vi "UHR-Fleezers Control (host) -Leonardo 04-2018 V2.vi"(0 "Tab Control":T5(tab)=enum."Trap Control (RF)") -> ()   [LabVIEW 2013] (continued)
        n1860 = call-poly <vilib>:"Mean.vi"("X"=w2816) -> ("mean"=w2803:dbl)  [unwired: 1 out]
        n1861 = call-poly <vilib>:"Mean.vi"("X"=w2815) -> ("mean"=w2801:dbl)  [unwired: 1 out]
        n1862 = call-poly <vilib>:"Mean.vi"("X"=w2779) -> ("mean"=w2770:dbl)  [unwired: 1 out]
        n1863 = Subtract(x=w2874, y=w2866) -> (x-y=w2808:u64)
        n1864 = call-poly <vilib>:"Mean.vi"("X"=w2864) -> ("mean"=w2805:dbl)  [unwired: 1 out]
        n1865 = Initialize Array(1.0 ("element"), w2773) -> (w2769:dbl[])
        n1866 = Initialize Array(1.0 ("element"), w2808) -> (w2799:dbl[])
        n1867 = Multiply(x=w2769, y=w2770) -> (x*y=w2771:dbl[])
        n1868 = Multiply(x=w2799, y=w2801) -> (x*y=w2802:dbl[])
        n1869 = Multiply(x=w2799, y=w2803) -> (x*y=w2804:dbl[])
        n1870 = Multiply(x=w2799, y=w2798) -> (x*y=w2800:dbl[])
        n1871 = Multiply(x=w2799, y=w2805) -> (x*y=w2806:dbl[])
        n1872 = Build Array (concatenate)(w2814, w2800) -> (w2868:dbl[])
        n1873 = Build Array (concatenate)(w2816, w2804) -> (w2872:dbl[])
        n1874 = Build Array (concatenate)(w2815, w2802) -> (w2871:dbl[])
        n1875 = Build Array (concatenate)(w2779, w2771) -> (w2781:dbl[])
        n1876 = Build Array (concatenate)(w2864, w2806) -> (w2873:dbl[])
        n1877 = Reshape Array(w2868, w2752, w2751) -> (w2834:dbl[][])
        n1878 = Reshape Array(w2781, w2752, w2751) -> (w2777:dbl[][])
        n1879 = Reshape Array(w2872, w2752, w2751) -> (w2826:dbl[][])
        n1880 = Reshape Array(w2871, w2752, w2751) -> (w2841:dbl[][])
        n1881 = Reshape Array(w2873, w2752, w2751) -> (w2851:dbl[][])
        n1882 = Array Subset(array=w2841, index (col)=0 ("index"), length (col)=w2766) -> (w2846:dbl[][])  [unwired: 2 in]
        n1883 = Array Subset(array=w2841, index (col)=w2766) -> (w2844:dbl[][])  [unwired: 3 in]
        n1884 = Array Subset(array=w2826, index (col)=0 ("index"), length (col)=w2766) -> (w2832:dbl[][])  [unwired: 2 in]
        n1885 = Array Subset(array=w2826, index (col)=w2766) -> (w2830:dbl[][])  [unwired: 3 in]
        n1886 = Array Subset(array=w2777, index (col)=0 ("index"), length (col)=w2766) -> (w2776:dbl[][])  [unwired: 2 in]
        n1887 = Array Subset(array=w2777, index (col)=w2766) -> (w2774:dbl[][])  [unwired: 3 in]
        n1888 = Array Subset(array=w2851, index (col)=0 ("index"), length (col)=w2766) -> (w2850:dbl[][])  [unwired: 2 in]
        n1889 = Array Subset(array=w2851, index (col)=w2766) -> (w2848:dbl[][])  [unwired: 3 in]
        n1890 = Array Subset(array=w2834, index (col)=0 ("index"), length (col)=w2766) -> (w2839:dbl[][])  [unwired: 2 in]
        n1891 = Array Subset(array=w2834, index (col)=w2766) -> (w2837:dbl[][])  [unwired: 3 in]
        n1892 = for {
          tunnel: w2846 -> [w2888] mode=indexing
          tunnel: [w2887] -> w2845 mode=indexing
          workers-P: _ -> [_]
          n1893 = Reverse 1D Array(array=w2888) -> (reversed array=w2887:dbl[])
        }
        n1894 = for {
          tunnel: w2832 -> [w2884] mode=indexing
          tunnel: [w2883] -> w2831 mode=indexing
          workers-P: _ -> [_]
          n1895 = Reverse 1D Array(array=w2884) -> (reversed array=w2883:dbl[])
        }
        n1896 = for {
          tunnel: w2776 -> [w2882] mode=indexing
          tunnel: [w2881] -> w2775 mode=indexing
          workers-P: _ -> [_]
          n1897 = Reverse 1D Array(array=w2882) -> (reversed array=w2881:dbl[])
        }
        n1898 = for {
          tunnel: w2850 -> [w2890] mode=indexing
          tunnel: [w2889] -> w2849 mode=indexing
          workers-P: _ -> [_]
          n1899 = Reverse 1D Array(array=w2890) -> (reversed array=w2889:dbl[])
        }
        n1900 = for {
          tunnel: w2839 -> [w2886] mode=indexing
          tunnel: [w2885] -> w2838 mode=indexing
          workers-P: _ -> [_]
          n1901 = Reverse 1D Array(array=w2886) -> (reversed array=w2885:dbl[])
        }
        n1902 = Index Array(array=w2851, index (row)=0) -> (element=→"Waveform Graph":dbl[])  [unwired: 1 in]
        n1903 = Add(x=w2845, y=w2844) -> (x+y=w2843:dbl[][])
        n1904 = Add(x=w2831, y=w2830) -> (x+y=w2829:dbl[][])
        n1905 = Add(x=w2775, y=w2774) -> (x+y=w2759:dbl[][])
        n1906 = Add(x=w2849, y=w2848) -> (x+y=w2823:dbl[][])
        n1907 = Add(x=w2838, y=w2837) -> (x+y=w2836:dbl[][])
        n1908 = Divide(x=w2829, y=2) -> (x/y=w2827:dbl[][])
        n1909 = Divide(x=w2843, y=2) -> (x/y=w2788:dbl[][])
        n1910 = Divide(x=w2836, y=2) -> (x/y=w2790:dbl[][])
        n1911 = To Single Precision Float(number=w2823) -> (single precision float=w2822:sgl[][])
        n1912 = Transpose 2D Array(2D array=w2827) -> (transposed array=→"Data map":dbl[][])
        n1913 = To Single Precision Float(number=w2759) -> (single precision float=w2763:sgl[][])
        n1914 = To Single Precision Float(number=w2788) -> (single precision float=w2794:sgl[][])
        n1915 = To Single Precision Float(number=w2790) -> (single precision float=w2791:sgl[][])
        n1916 = call "IMAQ ArrayToImage"("Image Pixels (Float)"=w2822, "Image"=w2756) -> ("Image Out"=w2825:T3)  [unwired: 8 in, 1 out]
        n1917 = call "IMAQ ArrayToImage"("Image Pixels (Float)"=w2763, "Image"=w2755) -> ("Image Out"=w2765:T3)  [unwired: 8 in, 1 out]
        n1918 = call "IMAQ ArrayToImage"("Image Pixels (Float)"=w2794, "Image"=w2754) -> ("Image Out"=w2796:T3)  [unwired: 8 in, 1 out]
        n1919 = call "IMAQ ArrayToImage"("Image Pixels (Float)"=w2791, "Image"=w2753) -> ("Image Out"=w2793:T3)  [unwired: 8 in, 1 out]
        n1920 = call "IMAQ Symmetry"("Type of Symmetry"=w2824, "Image Src"=w2825) -> ("Image Dst Out"=w2820:T3)  [unwired: 3 in, 1 out]
        n1921 = call "IMAQ Symmetry"("Type of Symmetry"=w2764, "Image Src"=w2765) -> ("Image Dst Out"=w2761:T3)  [unwired: 3 in, 1 out]
        n1922 = call "IMAQ Symmetry"("Type of Symmetry"=w2795, "Image Src"=w2796) -> ("Image Dst Out"=→"Detection Laser X":T3)  [unwired: 3 in, 1 out]
        n1923 = call "IMAQ Symmetry"("Type of Symmetry"=w2792, "Image Src"=w2793) -> ("Image Dst Out"=→"Detection Laser Y":T3)  [unwired: 3 in, 1 out]
        n1924 = call "IMAQ Set Simple Calibration"("Calibration Axis Info"=T37 {"Origin Pixel"={"X"=0.0, "Y"=0.0}, "Angle Relative to Horizontal (deg)"=0.0, "Axis Reference"=0}, "Grid Descriptor"=T38 {"X Step"=0.3, "Y Step"=0.3, "Unit"=enum."Undefined"}, "Image"=w2820) -> ("Calibrated Image"=→"APD 1":T3)  [unwired: 7 in, 1 out]
        n1925 = call "IMAQ Set Simple Calibration"("Calibration Axis Info"=T37 {"Origin Pixel"={"X"=0.0, "Y"=0.0}, "Angle Relative to Horizontal (deg)"=0.0, "Axis Reference"=0}, "Grid Descriptor"=T38 {"X Step"=0.3, "Y Step"=0.3, "Unit"=enum."Undefined"}, "Image"=w2761) -> ("Calibrated Image"=→"APD 2":T3)  [unwired: 7 in, 1 out]
      }
    }
    n1926 = Subtract(x=w2303, y="APD 2 Offset") -> (x-y=w2300:waveform(dbl))
    n1927 = Subtract(x=w2305, y="APD 1 Offset") -> (x-y=w2301:waveform(dbl))
    n1928 = Index Array(array=w2320, index=3) -> (element=w2379:waveform(dbl))
    n1929 = Index Array(array=w2320, index=6) -> (element=w2376:waveform(dbl))
    n1930 = Build Array(w2301, w2300) -> (→"APD Chart":waveform(dbl)[])
    n1931 = Array Size(array=w2369) -> (size(s)=w2417:i32)
    n1932 = call <vilib>:"Std Deviation and Variance.vi"("X"=w2313) -> ("standard deviation"=w2312:dbl)  [unwired: 1 in, 2 out]
    n1933 = Add Array Elements(numeric array=w2313) -> (sum=w2315:u32)
    n1934 = Add Array Elements(numeric array=w2369) -> (sum=w2427:u32)
    n1935 = call <vilib>:"Std Deviation and Variance.vi"("X"=w2369) -> ("standard deviation"=w2368:dbl)  [unwired: 1 in, 2 out]
    n1936 = Divide(x=w2312, y=w2311) -> (x/y=w2308:dbl)
    "Rate sigma (Hz) 2" <- w2308
    n1937 = Multiply(x=w2311, y=w2417) -> (x*y=w2314:dbl)
    "Int. Time (s)" <- w2314
    n1938 = Divide(x=w2315, y=w2314) -> (x/y=w2309:dbl)
    "APD 2 Rate (Hz)" <- w2309
    n1939 = Divide(x=w2427, y=w2314) -> (x/y=w2366:dbl)
    "APD 1 Rate (Hz)" <- w2366
    n1940 = Divide(x=w2368, y=w2311) -> (x/y=w2367:dbl)
    "Rate sigma (Hz)" <- w2367
    n1941 = Divide(x=w2308, y=w2309) -> (x/y=→"Sigma/Mean 2":dbl)
    n1942 = Divide(x=w2367, y=w2366) -> (x/y=→"Sigma/Mean":dbl)
    n1943 = case shown="2" "Calibration" {
      tunnel: "T1 alpha_x (nm/V)" -> [_ w2719 w2740]
      tunnel: "T1 kappa_x (pN/nm)" -> [_ _ w2730]
      tunnel: "T2 alpha_x (nm/V)" -> [_ w2718 w2738]
      tunnel: "T2 kappa_x (pN/nm)" -> [_ _ w2731]
      tunnel: w2379 -> [w2701 w2716 w2736]
      tunnel: w2376 -> [w2700 w2714 w2734]
      tunnel: [w2701 w2713 w2733] -> w2169
      tunnel: [w2700 w2712 w2732] -> w2175
      tunnel: ["T1 X (V)" ("Label.Text") "T1 X (nm)" ("Label.Text") "T1 X (pN)" ("Label.Text")] -> w2397
      tunnel: ["T2 X (V)" ("Label.Text") "T2 X (nm)" ("Label.Text") "T2 X (pN)" ("Label.Text")] -> w2396
      tunnel: ["Position (V)" ("Label.Text") "Position (nm)" ("Label.Text") "Force (pN)" ("Label.Text")] -> w2398
      tunnel: w2378 -> [_ w2704 w2723]
      tunnel: w2380 -> [_ w2707 w2725]
      tunnel: ["Mean (V)" ("Label.Text") "Mean (nm)" ("Label.Text") "Mean (pN)" ("Label.Text")] -> w2393
      tunnel: ["Difference (V)" ("Label.Text") "Difference (nm)" ("Label.Text") "Difference (pN)" ("Label.Text")] -> w2328
      frame 0, Default {
      }
      frame 1 {
        # "position"
        n1944 = Unbundle By Name(w2716) -> ("Y"=w2720:dbl[])
        n1945 = Unbundle By Name(w2714) -> ("Y"=w2705:dbl[])
        n1946 = Subtract(x=w2720, y=w2707) -> (x-y=w2708:dbl[])
        n1947 = Subtract(x=w2705, y=w2704) -> (x-y=w2706:dbl[])
        n1948 = Multiply(x=w2706, y=w2718) -> (x*y=w2715:dbl[])
        n1949 = Multiply(x=w2719, y=w2708) -> (x*y=w2717:dbl[])
        n1950 = Bundle By Name(cluster=w2714, "Y"=w2715) -> (w2712:waveform(dbl))
        n1951 = Bundle By Name(cluster=w2716, "Y"=w2717) -> (w2713:waveform(dbl))
      }
      frame 2 {
        # "force"
        n1952 = Unbundle By Name(w2736) -> ("Y"=w2741:dbl[])
        n1953 = Unbundle By Name(w2734) -> ("Y"=w2739:dbl[])
        n1954 = Subtract(x=w2739, y=w2723) -> (x-y=w2724:dbl[])
        n1955 = Subtract(x=w2741, y=w2725) -> (x-y=w2726:dbl[])
        n1956 = Compound Arithmetic op=MULTIPLY(w2724, w2738, w2731) -> (w2735:dbl[])
        n1957 = Compound Arithmetic op=MULTIPLY(w2730, w2740, w2726) -> (w2737:dbl[])
        n1958 = Bundle By Name(cluster=w2734, "Y"=w2735) -> (w2732:waveform(dbl))
        n1959 = Bundle By Name(cluster=w2736, "Y"=w2737) -> (w2733:waveform(dbl))
      }
    }
    n1960 = feedback-in #17("Calibration") -> ()
    n1961 = feedback #17(u16 1 ("Calibration")) -> (w2400:u16)
    n1962 = local read "Trap 2 Bead Size (nm)"() -> (w2208:dbl)
    n1963 = local read "Trap 1 Bead Size (nm)"() -> (w2207:dbl)
    n1964 = local read "AOM X Cal (nm/MHz)"() -> (w2205:dbl)
    n1965 = local read "Trap Delta (MHz)"() -> (w2204:dbl)
    n1966 = Not Equal?(x=w2400, y="Calibration") -> (x != y?=w2357:bool)
    n1967 = Multiply(x=w2205, y=w2204) -> (x*y=w2209:dbl)
    n1968 = Unbundle By Name(w2169) -> ("Y"=w2174:dbl[])
    n1969 = Unbundle By Name(w2175) -> ("Y"=w2173:dbl[])
    n1970 = Add(x=w2208, y=w2207) -> (x+y=w2211:dbl)
    n1971 = case shown="False" "Negate trap 2 force" {
      tunnel: [-1.0 1.0] -> w2386
      frame False {
      }
      frame True {
      }
    }
    n1972 = Unbundle By Name(w2379) -> ("Y"=w2382:dbl[])
    n1973 = Unbundle By Name(w2376) -> ("Y"=w2385:dbl[])
    n1974 = Divide(x=w2211, y=2.0) -> (x/y=w2206:dbl)
    n1975 = Subtract(x=w2174, y=w2173) -> (x-y=w2171:dbl[])
    n1976 = Subtract(x=w2382, y=w2380) -> (x-y=w2383:dbl[])
    n1977 = Subtract(x=w2385, y=w2378) -> (x-y=w2384:dbl[])
    n1978 = Divide(x=w2171, y=2.0) -> (x/y=w2170:dbl[])
    n1979 = Multiply(x=w2384, y="T2 alpha_x (nm/V)") -> (x*y=w2375:dbl[])
    n1980 = Multiply(x="T1 alpha_x (nm/V)", y=w2383) -> (x*y=w2374:dbl[])
    n1981 = Multiply(x=w2175, y=w2386) -> (x*y=w2387:waveform(dbl))
    n1982 = Bundle By Name(cluster=w2169, "Y"=w2170) -> (w2168:waveform(dbl))
    n1983 = case shown="True" "Read Lateness and Rel Phase" {
      tunnel: w2181 -> [w2665 w2689]
      tunnel: w2220 -> [w2666 w2688]
      tunnel: [w2665 w2687] -> w2372
      tunnel: [w2666 w2686] -> w2371
      frame False {
      }
      frame True {
        n1984 = xnode "Read/Write Control"("FPGA VI Reference In"=w2689, "error in"=w2688) -> ("FPGA VI Reference Out"=w2687:T20, "error out"=w2686:errorcluster, "GI Relative phase"=→"GI relative phase":i16, "Relative phase"=→"Relative phase (AI1)":i16, "AI Late Counter"=→"Late Counter (AI1)":u8, "GI Late Counter"=→"GI Late Counter":u8, "MCL Late Counter"=→"MCL Late Counter":u8, "MCL Relative Phase"=→"Relative Phase (MCL)":i16, "APD Acq Relative Phase"=→"APD Acq Relative Phase":i16, "APD 1 Gate Relative Phase"=→"APD 1 Gate Relative Phase":i16, "APD Acq Late Counter"=→"APD Acq Late Counter":u16, "APD 1 Gate Late Counter"=→"APD 1 Gate Late Counter":u8, "Green FB Relative Phase"=→"Relative phase (Green FB)":i16, "GI Relative phase"=→"GI relative phase 2":i16, "GI Late Counter 2"=→"GI Late Counter 2":u16, "Trap Pos FIFO Timeout"=→"Trap Pos FIFO Timeout":u16, "Trap AI FIFO Timeout"=→"Trap AI FIFO Timeout":u16, "APD 1 Counts 0"=→"APD1 counts 1":u32, "APD 1 Counts 1"=→"APD1 counts 2":u32, "APD 2 Counts 0"=→"APD2 counts 1":u32, "APD 2 Counts 1"=→"APD2 counts 2":u32)
      }
    }
    n1985 = Subtract(x=w2375, y=w2374) -> (x-y=w2203:dbl[])
    n1986 = call-poly <vilib>:"Mean.vi"("X"=w2203) -> ("mean"=w2210:dbl)  [unwired: 1 out]
    n1987 = Add(x=w2209, y=w2210) -> (x+y=w2213:dbl)
    n1988 = Subtract(x=w2213, y=w2206) -> (x-y=→"Tether Extension (nm, calculated)":dbl)
    n1989 = Unbundle By Name(w2175) -> ("Y"=w2166:dbl[])
    n1990 = Unbundle By Name(w2169) -> ("Y"=w2167:dbl[])
    n1991 = Build Array(w2169, w2387, w2168) -> (→"Force":waveform(dbl)[])
    n1992 = Subtract(x=w2203, y="Offset (nm)") -> (x-y=w2347:dbl[])
    n1993 = call-poly <vilib>:"Mean.vi"("X"=w2166) -> ("mean"=w2164:dbl)  [unwired: 1 out]
    "T2 X" <- w2164
    n1994 = call-poly <vilib>:"Mean.vi"("X"=w2167) -> ("mean"=w2165:dbl)  [unwired: 1 out]
    "T1 X" <- w2165
    n1995 = Subtract(x=w2167, y=w2166) -> (x-y=w2349:dbl[])
    n1996 = Bundle By Name(cluster=w2379, "Y"=w2347) -> (w2319:waveform(dbl))
    "Bead Separation" <- w2319
    n1997 = Divide(x=w2349, y=2.0) -> (x/y=→"Vec Mean of T1 T2":dbl[])
    n1998 = case shown="True" w2357 {
      tunnel: w2398 -> [_ w2694]
      tunnel: w2397 -> [_ w2693]
      tunnel: w2396 -> [_ w2692]
      tunnel: w2393 -> [_ w2691]
      tunnel: w2328 -> [_ w2690]
      frame False {
      }
      frame True {
        n1999 = property on="Force" class="WFChart (strict)"("YScale.NameLbl.Text"=w2694) -> ()  [unwired: 2 in, 2 out]
        n2000 = property on="T2 X" class="DigNum (strict)"("Caption.Text"=w2692) -> ()  [unwired: 2 in, 2 out]
        n2001 = property on="T1 X" class="DigNum (strict)"("Caption.Text"=w2693) -> ()  [unwired: 2 in, 2 out]
        n2002 = property on="Mean" class="DigNum (strict)"("Caption.Text"=w2691) -> ()  [unwired: 2 in, 2 out]
        n2003 = property on="Difference" class="DigNum (strict)"("Caption.Text"=w2690) -> ()  [unwired: 2 in, 2 out]
      }
    }
    n2004 = local read "Tether"() -> (w2351:bool)
    n2005 = Subtract(x=w2165, y=w2164) -> (x-y=w2395:dbl)
    n2006 = Add(x=w2165, y=w2164) -> (x+y=→"Difference":dbl)
    n2007 = feedback #18(w2347) -> (w2346:dbl[])
    n2008 = Divide(x=w2395, y=2.0) -> (x/y=w2178:dbl)
    "Mean" <- w2178
    n2009 = case shown="True" w2351 {
      tunnel: w2178 -> [_ w2624]
      frame False {
      }
      frame True {
        n2010 = Greater?(x="Lost Tether Alarm Threshold (pN)", y=w2624) -> (0:w2622:bool)
        n2011 = case shown="True" w2622 {
          frame False {
          }
          frame True {
            n2012 = flat-sequence {
              frame #0 {
                # "stop only if saving"
                n2013 = local read "Saving..."() -> (w2637:bool)
                n2014 = And(x=w2637, y="TA Cancel Save?") -> (x .and. y?=w2636:bool)
                n2015 = local write "Stop Saving"(w2636) -> ()
              }
              frame #1 {
                n2016 = case shown="True" "TA Green Off?" {
                  frame False {
                  }
                  frame True {
                    w2640 = FALSE ("Fl. Triggered...")
                    n2017 = local write "Fl. Triggered..."(w2640) -> ()
                    n2018 = property on="Green Laser ON/Interlacing" class="Bool (strict)"("Val(Sgnl)"=w2640) -> ()  [unwired: 2 in, 2 out]
                  }
                }
              }
            }
            n2019 = local read "Time tether formed"() -> (w2631:timestamp)
            n2020 = Get Date/Time In Seconds() -> (seconds since 1Jan1904=w2632:timestamp)
            n2021 = Subtract(x=w2632, y=w2631) -> (x-y=w2630:dbl)
            n2022 = Number To Decimal String(number=w2630) -> (decimal integer string=w2627:string)  [unwired: 1 out]
            n2023 = local read "Messages"() -> (w2634:string)
            n2024 = call <vilib>:"Beep.vi"() -> ()  [unwired: 3 in, 9 out]
            n2025 = Concatenate Strings("Lost tether (" ("Message to add"), w2627, " s)." ("string")) -> (w2629:string)
            n2026 = local write "Tether"(FALSE ("Tether")) -> ()
            n2027 = call "Update messages.vi"("Message to add"=w2629, "Old message string"=w2634) -> ("New message string"=w2633:string)
            n2028 = local write "Messages"(w2633) -> ()
            n2029 = property on="Trap Pos. FB ON" class="Bool (strict)"("Val(Sgnl)"=FALSE ("Value (Signaling)")) -> ()  [unwired: 2 in, 2 out]
          }
        }
      }
    }
    n2030 = Build Array (concatenate)(w2347, w2346) -> (w2345:dbl[])
    n2031 = Split 1D Array(array=w2345, index=w2231) -> (first subarray=w2341:dbl[])  [unwired: 1 out]
    n2032 = feedback-in #18(w2341) -> ()
    n2033 = call-poly <vilib>:"Mean.vi"("X"=w2341) -> ("mean"=w2340:dbl)  [unwired: 1 out]
    "Bead Mean (nm)" <- w2340
    n2034 = Subtract(x=w2341, y=w2340) -> (x-y=w2339:dbl[])
    n2035 = Square(x=w2339) -> (x^2=w2338:dbl[])
    n2036 = call-poly <vilib>:"Mean.vi"("X"=w2338) -> ("mean"=w2337:dbl)  [unwired: 1 out]
    n2037 = case shown="True" "Semi Passive ON" {
      tunnel: "Semi Passive mode" -> [_ w2505]
      tunnel: "Jump Force (pN)" -> [_ w2504]
      tunnel: w2178 -> [_ w2503]
      frame False {
      }
      frame True {
        n2038 = case shown="\"Use Feedback\"" w2505 {
          tunnel: w2504 -> [_ w2508 w2524]
          tunnel: w2503 -> [_ w2507 w2523]
          frame "None" {
          }
          frame "Use Feedback" {
            n2039 = local read "Target Force (pN)"() -> (w2510:dbl)
            n2040 = Less?(x=w2508, y=w2510) -> (x < y?=w2509:bool)
            n2041 = case shown="True" w2509 {
              tunnel: w2508 -> [w2517 w2520]
              tunnel: w2507 -> [w2516 w2519]
              tunnel: [w2515 w2518] -> w2506
              frame False {
                n2042 = Less?(x=w2517, y=w2516) -> (x < y?=w2515:bool)
              }
              frame True {
                n2043 = Greater?(x=w2520, y=w2519) -> (0:w2518:bool)
              }
            }
            n2044 = case shown="True" w2506 {
              frame False {
                n2045 = local read "Trap Pos. FB ON"() -> (w2511:bool)
                n2046 = case shown="True" w2511 {
                  frame False {
                  }
                  frame True {
                    n2047 = property on="Trap Pos. FB ON" class="Bool (strict)"("Val(Sgnl)"=FALSE) -> ()  [unwired: 2 in, 2 out]
                  }
                }
              }
              frame True {
                n2048 = local read "Trap Pos. FB ON"() -> (w2513:bool)
                n2049 = case shown="False" w2513 {
                  frame False {
                    n2050 = property on="Trap Pos. FB ON" class="Bool (strict)"("Val(Sgnl)"=TRUE) -> ()  [unwired: 2 in, 2 out]
                  }
                  frame True {
                  }
                }
              }
            }
          }
          frame "Sharp Jump" {
            n2051 = local read "Target Force (pN)"() -> (w2526:dbl)
            n2052 = Greater?(x=w2524, y=w2526) -> (0:w2525:bool)
            n2053 = case shown="True" w2525 {
              tunnel: w2524 -> [w2541 w2545]
              tunnel: w2523 -> [w2542 w2544]
              tunnel: [w2540 w2543] -> w2522
              frame False {
                n2054 = Greater?(x=w2542, y=w2541) -> (0:w2540:bool)
              }
              frame True {
                n2055 = Less?(x=w2545, y=w2544) -> (x < y?=w2543:bool)
              }
            }
            n2056 = Subtract(x=w2524, y=w2526) -> (x-y=w2521:dbl)
            n2057 = case shown="True" w2522 {
              tunnel: w2521 -> [_ w2532]
              frame False {
              }
              frame True {
                n2058 = local read "T1 kappa_x (pN/nm)"() -> (w2537:dbl)
                n2059 = local read "T2 kappa_x (pN/nm)"() -> (w2538:dbl)
                n2060 = Reciprocal(x="DNA stiffness (pN / nm)") -> (1/x=w2534:dbl)
                n2061 = Reciprocal(x=w2537) -> (1/x=w2536:dbl)
                n2062 = Reciprocal(x=w2538) -> (1/x=w2535:dbl)
                n2063 = Compound Arithmetic op=ADD(w2536, w2535, w2534) -> (w2533:dbl)
                n2064 = local read "AOM X Cal (nm/MHz)"() -> (w2531:dbl)
                n2065 = Multiply(x=w2533, y=w2532) -> (x*y=w2530:dbl)
                n2066 = local read "Trap Delta (MHz)"() -> (w2528:dbl)
                n2067 = Divide(x=w2530, y=w2531) -> (x/y=w2529:dbl)
                n2068 = Subtract(x=w2528, y=w2529) -> (x-y=w2527:dbl)
                n2069 = property on="Trap Delta (MHz)" class="DigNum (strict)"("Val(Sgnl)"=w2527) -> ()  [unwired: 2 in, 2 out]
              }
            }
          }
        }
      }
    }
    n2070 = Square Root(x=w2337) -> (sqrt(x)=w2336:dbl)
    n2071 = Multiply(x=10.0, y=w2336) -> (x*y=→"RMS (Ang)":dbl)
    n2072 = xnode "Read/Write Control"("FPGA VI Reference In"=w2372, "error in"=w2371) -> ("FPGA VI Reference Out"=w2481:T20, "error out"=w2475:errorcluster, "AI2 Y Sum Set 1"=w2471:i16, "AI2 Y Sum Set 2"=w2470:i16, "AI1 X Set 1"=w2265:fxp<+/-,16,1>, "AI1 X Set 2"=w2264:fxp<+/-,16,1>, "Trap Pos FB Int Signal"=→"Trap Pos FB Int Signal":fxp<+/-,24,9>, "Trap Pos FB Int-Norm Signal"=→"Trap Pos FB Int-Norm Signal":fxp<+/-,16,1>, "Trap Pos FB Action"=w2258:i64, "Scanning"=→"AOD Scanning":bool, "Scan I"=→"AOD Scan I":u64, "Scanning MCL"=w2473:bool, "Scan I (MCL)"=→"MCL Scan I":u64, "Green FB Signals"=w2412:T48, "BD1 amplitude 1 out"=w2163:u16, "BD1 amplitude 2 out"=w2148:u16)  [unwired: 1 out]
    "MCL Scanning" <- w2473
    "Trap Pos FB Action" <- w2258
    n2073 = local read "AI2 (V)"() -> (w2472:cluster{"Set 1":dbl, "Set 2":dbl})
    n2074 = Bundle By Name(cluster=w2472, "Set 1"=w2471, "Set 2"=w2470) -> (w2468:cluster{"Set 1":dbl, "Set 2":dbl})
    n2075 = Divide(x=w2258, y=327.67) -> (x/y=→"Action (%)":dbl)
    n2076 = local read "Trap X (AI1)"() -> (w2278:T1)
    n2077 = Divide(x=w2468, y=3276.7) -> (x/y=w2467:cluster{"Set 1":dbl, "Set 2":dbl})
    n2078 = local write "AI2 (V)"(w2467) -> ()
    n2079 = Bundle(cluster=w2278, "Trap 1"=w2265, "Trap 2"=w2264) -> (→"Trap X (AI1)":T1)
    n2080 = Scale By Power Of 2(n=i16 12, x=ext 1.0) -> (x*2^n=w2159:ext)
    n2081 = Subtract(x=w2159, y=ext 1.0) -> (x-y=w2156:ext)
    n2082 = Divide(x=w2412, y=3276.7) -> (x/y=w2408:T49)
    n2083 = Multiply(x=w2163, y=ext 100.0) -> (x*y=w2157:ext)
    n2084 = Unbundle By Name(w2408) -> ("Green FB Ch 0"=w2411:dbl, "Green FB Ch 1"=w2410:dbl, "Green FB Ch 2"=w2409:dbl)
    n2085 = local read "All FB On/Off"() -> (w2147:bool)
    n2086 = Divide(x=w2157, y=w2156) -> (x/y=w2146:ext)
    "Trap 1 amplitude" <- w2146
    n2087 = Scale By Power Of 2(n=i16 12, x=ext 1.0) -> (x*2^n=w2152:ext)
    n2088 = Subtract(x=w2152, y=ext 1.0) -> (x-y=w2155:ext)
    n2089 = Multiply(x=w2148, y=ext 100.0) -> (x*y=w2154:ext)
    n2090 = Divide(x=w2411, y=w2409) -> (x/y=w2407:dbl)
    n2091 = Divide(x=w2410, y=w2409) -> (x/y=w2406:dbl)
    n2092 = flat-sequence "To save data" {
      tunnel: [w3521] -> w2492
      tunnel: [w3522] -> w2491
      tunnel: w2443 -> [w3515]
      tunnel: w2343 -> [w3519]
      tunnel: ["Save Calibration"] -> w2464
      tunnel: w2461 -> [w3518]
      tunnel: [w3511] -> w2460
      tunnel: [w3508] -> w2459
      tunnel: [w3505] -> w2458
      tunnel: w2442 -> [w3507]
      tunnel: w2355 -> [w3501]
      tunnel: [w3501] -> w2354
      tunnel: ["Start Saving"] -> w2321
      tunnel: [w3495] -> w2247
      tunnel: [w3494] -> w2246
      tunnel: w2492 -> [w3756]
      tunnel: w2491 -> [w3755]
      tunnel: w2248 -> [w3754]
      tunnel: w2464 -> [w3753]
      tunnel: w2460 -> [w3751]
      tunnel: w2459 -> [w3750]
      tunnel: w2458 -> [w3749]
      tunnel: w2330 -> [w3748]
      tunnel: w2364 -> [w3747]
      tunnel: w2354 -> [w3746]
      tunnel: w2321 -> [w3745]
      tunnel: w2319 -> [w3744]
      tunnel: w2295 -> [w3743]
      tunnel: w2247 -> [w3742]
      tunnel: w2246 -> [w3741]
      tunnel: w2245 -> [w3740]
      frame #0 {
        n2093 = Or(x="Save N Sets", y="Start Saving") -> (x .or. y?=w3502:bool)
        n2094 = To Double Precision Float(number=w3518) -> (double precision float=w3512:dbl)
        n2095 = Build Array(w3502, "Save Calibration", w3515, w3507) -> (w3517:bool[])
        n2096 = Compound Arithmetic op=OR("Save Calibration", w3515, w3502, w3507) -> (w3520:bool)
        n2097 = Boolean Array To Number(Boolean array=w3517) -> (number=w3514:u32)
        n2098 = feedback #19(FALSE ("Save APD Data\nwith Trap Data")) -> (w3496:bool)
        n2099 = feedback #20(refnum<k0> refnum) -> (w3523:refnum<file>)
        n2100 = feedback #21(refnum<k0> refnum) -> (w3498:refnum<file>)
        n2101 = feedback #22(FALSE ("Save APD Data\nwith Trap Data")) -> (w3506:bool)
        n2102 = feedback #23(refnum<k0> refnum) -> (w3509:refnum<file>)
        n2103 = feedback #24(0) -> (w3525:i32)
        n2104 = feedback #25() -> (w3513:u32)  [unwired: 1 out]
        n2105 = case shown="True" w3520 {
          tunnel: [w3532 1] -> w3521
          tunnel: w3525 -> [w3534 _]
          tunnel: [w3533 w3552] -> w3522
          tunnel: w3523 -> [w3533 _]
          tunnel: w3519 -> [_ w3572]
          tunnel: w3512 -> [_ w3570]
          tunnel: w3514 -> [_ w3573]
          tunnel: [w3531 w3551] -> w3511
          tunnel: w3513 -> [w3531 _]
          tunnel: [w3530 w3549] -> w3508
          tunnel: w3509 -> [w3530 _]
          tunnel: [w3529 w3548] -> w3505
          tunnel: w3506 -> [w3529 _]
          tunnel: "Start Saving" -> [_ w3546]
          tunnel: w3501 -> [_ w3545]
          tunnel: [w3528 w3536] -> w3494
          tunnel: w3498 -> [w3528 _]
          tunnel: [w3527 w3535] -> w3495
          tunnel: w3496 -> [w3527 _]
          frame False {
            n2106 = Increment(x=w3534) -> (x+1=w3532:i32)
          }
          frame True {
            w3542 = FALSE ("Start Saving")
            w3547 = 9.0  # File Version
            w3555 = FALSE ("prepend array or string size? (T)")
            w3553 = T30."big-endian, network order" ("byte order (0:big-endian, network order)")
            # "write file headers"
            n2107 = local read "BD 1 Frequency 1 (MHz)"() -> (w3569:dbl)
            n2108 = local read "BD 2 Frequency 1 (MHz)"() -> (w3568:dbl)
            n2109 = local read "BD 1 Frequency 2 (MHz)"() -> (w3567:dbl)
            n2110 = local read "BD 2 Frequency 2 (MHz)"() -> (w3566:dbl)
            n2111 = local read "BD 1 Frequency 3 (MHz)"() -> (w3565:dbl)
            n2112 = local read "BD 2 Frequency 3 (MHz)"() -> (w3564:dbl)
            n2113 = Array Size(array=w3545) -> (size(s)=w3544:i32)
            n2114 = To Double Precision Float(number=w3544) -> (double precision float=w3543:dbl)
            n2115 = local write "Save Calibration"(w3542) -> ()
            n2116 = local write "Start Saving"(w3542) -> ()
            n2117 = Build Array("Save APD Data\nwith Trap Data", "Save Trap Pos. Data") -> (w3539:bool[])
            n2118 = Boolean Array To Number(Boolean array=w3539) -> (number=w3538:u32)
            n2119 = Build Array(w3569, w3568, w3567, w3566, w3565, w3564) -> (w3563:dbl[])
            n2120 = case shown="4" w3573 {
              tunnel: w3572 -> [w3644 w3664 w3680 w3718]
              tunnel: w3543 -> [w3649 w3671 w3700 w3737]
              tunnel: w3570 -> [w3648 w3670 w3699 w3736]
              tunnel: [w3645 w3666 w3691 w3728] -> w3561
              tunnel: [w3636 "Cal sets to save" w3681 w3719] -> w3551
              tunnel: w3563 -> [w3646 w3667 w3693 w3730]
              tunnel: "Save APD Data\nwith Trap Data" -> [w3643 _ w3677 w3716]
              tunnel: [w3643 w3658 w3677 w3716] -> w3548
              tunnel: w3547 -> [w3639 w3659 w3675 w3714]
              tunnel: w3546 -> [w3638 _ _ _]
              tunnel: [w3629 w3658 w3674 w3704] -> w3535
              tunnel: "Save Trap Pos. Data" -> [w3629 _ w3674 w3704]
              tunnel: w3538 -> [w3628 _ w3673 w3703]
              frame 1, Default {
                # "timeseries"
                n2121 = case shown="True" "Profile" {
                  tunnel: [w3652 w3655] -> w3633
                  tunnel: [w3652 w3654] -> w3632
                  tunnel: [w3652 w3653] -> w3631
                  tunnel: [w3652 w3657] -> w3630
                  frame False {
                    w3652 = 0.0 ("f")
                  }
                  frame True {
                    n2122 = local read "Current Position"() -> (w3656:dbl[])
                    n2123 = local read "Y change (mm)"() -> (w3657:dbl)
                    n2124 = call "subVI_explode3array.vi"("Array"=w3656) -> ("x"=w3655:dbl, "y"=w3654:dbl, "z"=w3653:dbl)  [unwired: 12 in]
                  }
                }
                n2125 = local read "Save ave N"() -> (w3651:dbl)
                n2126 = Multiply(x=w3651, y=w3644) -> (x*y=w3650:dbl)
                n2127 = To Double Precision Float(number=w3628) -> (double precision float=w3642:dbl)
                n2128 = Build Array(w3639, w3644, w3650, w3649, w3648, 0.0 ("f")) -> (w3647:dbl[])
                n2129 = Build Array(w3642, w3633, w3632, w3631, w3630) -> (w3640:dbl[])
                n2130 = Select(t=u32 4000000000, s=w3638, f="N sets to save") -> (s? t:f=w3636:u32)
                n2131 = Build Array (concatenate)(w3647, w3646, w3640) -> (w3645:dbl[])
              }
              frame 2 {
                w3661 = 0.0 ("f")
                w3658 = FALSE ("Save APD Data\nwith Trap Data")
                # "calibration"
                n2132 = Boolean To (0,1)(Boolean=w3658) -> (0, 1=w3663:i16)
                n2133 = To Double Precision Float(number=w3663) -> (double precision float=w3662:dbl)
                n2134 = Build Array(w3662, w3661, w3661, w3661, w3661) -> (w3660:dbl[])
                n2135 = Build Array(w3659, w3664, w3664, w3671, w3670, 1.0 ("t")) -> (w3668:dbl[])
                n2136 = Build Array (concatenate)(w3668, w3667, w3660) -> (w3666:dbl[])
                "Calibrating Trap..." <- TRUE ("Calibrating...")
              }
              frame 4 {
                w3678 = 0.0 ("f")
                # "write file header for a trap \nraster scan"
                # "scan dir (x/y = 0/1)"
                # "cycles/step"
                # "n scans (f/b)"
                # "steps"
                # "freq. range"
                # "AOD raster scan"
                n2137 = local read "Number of F/B Scans (AOD)"() -> (w3685:u16)
                n2138 = local read "Cycles/step (AOD)"() -> (w3687:u64)
                n2139 = local read "Scan Range (MHz)"() -> (w3690:dbl)
                n2140 = local read "Scan steps (AOD)"() -> (w3689:u64)
                n2141 = local read "Scan BD"() -> (w3697:bool)
                n2142 = local read "Save ave N"() -> (w3702:dbl)
                n2143 = Boolean To (0,1)(Boolean=w3697) -> (0, 1=w3696:i16)
                n2144 = To Double Precision Float(number=w3685) -> (double precision float=w3684:dbl)
                n2145 = To Double Precision Float(number=w3689) -> (double precision float=w3688:dbl)
                n2146 = To Double Precision Float(number=w3687) -> (double precision float=w3686:dbl)
                n2147 = To Double Precision Float(number=w3696) -> (double precision float=w3695:dbl)
                n2148 = Multiply(x=w3702, y=w3680) -> (x*y=w3701:dbl)
                n2149 = To Double Precision Float(number=w3673) -> (double precision float=w3679:dbl)
                n2150 = Build Array(w3679, w3678, w3678, w3678, w3678) -> (w3676:dbl[])
                n2151 = local read "N sets should be saved"() -> (w3682:dbl)
                n2152 = Build Array(w3695, w3690, w3688, w3686, w3684) -> (w3692:dbl[])
                n2153 = Build Array(w3675, w3680, w3701, w3700, w3699, 2.0 ("t")) -> (w3694:dbl[])
                n2154 = Round Toward +Infinity(x=w3682) -> (ceil(x): smallest int >= x=w3683:dbl)
                n2155 = Build Array (concatenate)(w3694, w3693, w3676, w3692) -> (w3691:dbl[])
                n2156 = To Unsigned Long Integer(number=w3683) -> (unsigned 32bit integer=w3681:u32)
              }
              frame 8 {
                w3711 = 0.0 ("f")
                # "MCL raster scan"
                n2157 = local read "Number of scans (MCL)"() -> (w3706:u64)
                n2158 = local read "Scan lines (y)"() -> (w3705:u64)
                n2159 = local read "2D or 1D Scan"() -> (w3708:bool)
                n2160 = local read "Scan Range (V)\n(of steps)"() -> (w3727:dbl)
                n2161 = local read "Fast Scan Dir"() -> (w3734:bool)
                n2162 = local read "Cycles/step (MCL)"() -> (w3724:u64)
                n2163 = local read "Scan steps (MCL)"() -> (w3726:u64)
                n2164 = Select(t=w3705, s=w3708, f=w3706) -> (s? t:f=w3707:u64)
                n2165 = Boolean To (0,1)(Boolean=w3708) -> (0, 1=w3710:i16)
                n2166 = local read "Save ave N"() -> (w3739:dbl)
                n2167 = local read "Initial X"() -> (w3713:dbl)
                n2168 = local read "Initial Y"() -> (w3712:dbl)
                n2169 = To Double Precision Float(number=w3710) -> (double precision float=w3709:dbl)
                n2170 = Boolean To (0,1)(Boolean=w3734) -> (0, 1=w3733:i16)
                n2171 = To Double Precision Float(number=w3707) -> (double precision float=w3722:dbl)
                n2172 = To Double Precision Float(number=w3726) -> (double precision float=w3725:dbl)
                n2173 = To Double Precision Float(number=w3724) -> (double precision float=w3723:dbl)
                n2174 = To Double Precision Float(number=w3733) -> (double precision float=w3732:dbl)
                n2175 = Multiply(x=w3739, y=w3718) -> (x*y=w3738:dbl)
                n2176 = To Double Precision Float(number=w3703) -> (double precision float=w3717:dbl)
                n2177 = local read "N sets should be saved (MCL)"() -> (w3720:dbl)
                n2178 = Build Array(w3717, w3709, w3711, w3711, w3711) -> (w3715:dbl[])
                n2179 = Build Array(w3732, w3727, w3725, w3723, w3722, w3713, w3712) -> (w3729:dbl[])
                n2180 = Build Array(w3714, w3718, w3738, w3737, w3736, 3.0 ("t")) -> (w3731:dbl[])
                n2181 = Round Toward +Infinity(x=w3720) -> (ceil(x): smallest int >= x=w3721:dbl)
                n2182 = Build Array (concatenate)(w3731, w3730, w3715, w3729) -> (w3728:dbl[])
                n2183 = To Unsigned Long Integer(number=w3721) -> (unsigned 32bit integer=w3719:u32)
              }
            }
            n2184 = local read "Index"() -> (w3578:dbl)
            n2185 = call "Create new save file.vi"("Insert"="", "Ext"=".dat", "Index In"=w3578) -> ("Path Out"=w3537:path, "Index Out"=w3550:dbl)
            n2186 = local write "Save file name"(w3537) -> ()
            n2187 = local write "Index"(w3550) -> ()
            n2188 = local write "Save index"(w3550) -> ()
            n2189 = Array Size(array=w3561) -> (size(s)=w3562:i32)
            n2190 = Open/Create/Replace File(file path (use dialog)=w3537, operation (0:open)=T24."create", access (0:read/write)=enum16{"read/write", "read-only", "write-only"}."write-only") -> (refnum out=w3575:refnum<file>)  [unwired: 1 in, 4 out]
            n2191 = local write "Saving..."(TRUE ("Saving...")) -> ()
            n2192 = To Double Precision Float(number=w3562) -> (double precision float=w3560:dbl)
            n2193 = String Length(string="Comment (data description)") -> (length=w3558:i32)
            n2194 = To Double Precision Float(number=w3558) -> (double precision float=w3557:dbl)
            n2195 = Deny Access(7:w3575) -> (3:w3574:refnum<file>)  [unwired: 1 in, 2 out]
            n2196 = Build Array (concatenate)(w3560, w3561, w3557) -> (w3559:dbl[])
            n2197 = case "If fluorescence data to be saved" shown="True" w3548 {
              tunnel: w3537 -> [_ w3627]
              tunnel: [refnum<k0> refnum w3607] -> w3549
              frame False {
              }
              frame True {
                w3606 = 0.0
                n2198 = local read "APD Integration Time (s)"() -> (w3612:dbl)
                n2199 = local read "N APD Samp/step"() -> (w3605:dbl)
                n2200 = Path To String(path=w3627) -> (string=w3626:string)
                n2201 = String Length(string=w3626) -> (length=w3625:i32)
                n2202 = Subtract(x=w3625, y=4) -> (x-y=w3623:i32)
                n2203 = String Subset(string=w3626, length (rest)=w3623) -> (substring=w3622:string)  [unwired: 1 out]
                n2204 = Build Array(w3612, w3605, w3606, w3606, w3606, w3606, w3606, w3606) -> (w3609:dbl[])
                n2205 = Concatenate Strings(w3622, "_fl.dat" ("string")) -> (w3620:string)
                n2206 = Array Size(array=w3609) -> (size(s)=w3611:i32)
                n2207 = String To Path(string=w3620) -> (path=w3616:path)
                n2208 = Open/Create/Replace File(file path (use dialog)=w3616, operation (0:open)=T24."create", access (0:read/write)=enum16{"read/write", "read-only", "write-only"}."write-only") -> (refnum out=w3617:refnum<file>)  [unwired: 1 in, 4 out]
                n2209 = Deny Access(7:w3617) -> (3:w3613:refnum<file>)  [unwired: 1 in, 2 out]
                n2210 = To Double Precision Float(number=w3611) -> (double precision float=w3610:dbl)
                n2211 = Build Array (concatenate)(w3610, w3609) -> (w3608:dbl[])
                n2212 = Write to Binary File(file (use dialog)=w3613, data=w3608, 5:FALSE ("prepend array or string size? (T)"), 9:T30."big-endian, network order" ("byte order (0:big-endian, network order)")) -> (refnum out=w3607:refnum<file>)  [unwired: 1 in, 3 out]
              }
            }
            n2213 = case shown="True" w3535 {
              tunnel: w3537 -> [_ w3589]
              tunnel: [refnum<k0> refnum w3588] -> w3536
              frame False {
              }
              frame True {
                w3584 = 0.0 ("element")
                n2214 = Path To String(path=w3589) -> (string=w3603:string)
                n2215 = Build Array(w3584, w3584, w3584, w3584, w3584, w3584, w3584, w3584) -> (w3585:dbl[])
                n2216 = String Length(string=w3603) -> (length=w3602:i32)
                n2217 = Subtract(x=w3602, y=4) -> (x-y=w3600:i32)
                n2218 = Array Size(array=w3585) -> (size(s)=w3587:i32)
                n2219 = String Subset(string=w3603, length (rest)=w3600) -> (substring=w3599:string)  [unwired: 1 out]
                n2220 = To Double Precision Float(number=w3587) -> (double precision float=w3586:dbl)
                n2221 = Concatenate Strings(w3599, "_pos.dat" ("string")) -> (w3597:string)
                n2222 = Build Array (concatenate)(w3586, w3585) -> (w3583:dbl[])
                n2223 = String To Path(string=w3597) -> (path=w3593:path)
                n2224 = Open/Create/Replace File(file path (use dialog)=w3593, operation (0:open)=T24."create", access (0:read/write)=enum16{"read/write", "read-only", "write-only"}."write-only") -> (refnum out=w3594:refnum<file>)  [unwired: 1 in, 4 out]
                n2225 = Deny Access(7:w3594) -> (3:w3590:refnum<file>)  [unwired: 1 in, 2 out]
                n2226 = Write to Binary File(file (use dialog)=w3590, data=w3583, 5:FALSE ("prepend array or string size? (T)"), 9:T30."big-endian, network order" ("byte order (0:big-endian, network order)")) -> (refnum out=w3588:refnum<file>)  [unwired: 1 in, 3 out]
              }
            }
            n2227 = Write to Binary File(file (use dialog)=w3574, data=w3559, 5:w3555, 9:w3553) -> (refnum out=w3556:refnum<file>)  [unwired: 1 in, 3 out]
            n2228 = Write to Binary File(file (use dialog)=w3556, data="Comment (data description)", 5:w3555, 9:w3553) -> (refnum out=w3552:refnum<file>)  [unwired: 1 in, 3 out]
          }
        }
        n2229 = feedback-in #19(w3495) -> ()
        n2230 = feedback-in #20(w3522) -> ()
        n2231 = feedback-in #21(w3494) -> ()
        n2232 = feedback-in #22(w3505) -> ()
        n2233 = feedback-in #23(w3508) -> ()
        n2234 = feedback-in #24(w3521) -> ()
        n2235 = feedback-in #25(w3511) -> ()
      }
      frame #1 {
        n2236 = local read "Saving..."() -> (w3752:bool)
        n2237 = case shown="True" w3752 {
          tunnel: w3756 -> [_ w3766]
          tunnel: w3755 -> [_ w3780]
          tunnel: w3754 -> [_ w3776]
          tunnel: w3753 -> [_ w3775]
          tunnel: w3751 -> [_ w3774]
          tunnel: w3750 -> [_ w3769]
          tunnel: w3749 -> [_ w3768]
          tunnel: w3748 -> [_ w3767]
          tunnel: w3747 -> [_ w3765]
          tunnel: w3746 -> [_ w3763]
          tunnel: w3745 -> [_ w3762]
          tunnel: w3744 -> [_ w3761]
          tunnel: w3743 -> [_ w3760]
          tunnel: w3742 -> [_ w3759]
          tunnel: w3741 -> [_ w3758]
          tunnel: w3740 -> [_ w3757]
          frame False {
          }
          frame True {
            n2238 = Multiply(x=w3766, y=w3765) -> (x*y=→"Time (s)":dbl)
            n2239 = Less Or Equal?(x=w3766, y=w3774) -> (x <= y?=w3778:bool)
            n2240 = Or(x="Stop Saving", y="Abort save 2") -> (x .or. y?=w3770:bool)
            n2241 = Not(x=w3770) -> (.not. x?=w3779:bool)
            n2242 = And(x=w3778, y=w3779) -> (x .and. y?=w3777:bool)
            n2243 = case shown="True" w3777 {
              tunnel: w3780 -> [w3787 w3855]
              tunnel: [0.0 w3858] -> w3773
              tunnel: w3766 -> [_ w3856]
              tunnel: w3774 -> [_ w3857]
              tunnel: w3776 -> [_ w3852]
              tunnel: w3775 -> [_ _]
              tunnel: w3769 -> [w3785 w3845]
              tunnel: w3768 -> [w3784 w3846]
              tunnel: w3767 -> [_ w3844]
              tunnel: w3763 -> [_ w3843]
              tunnel: w3762 -> [_ w3797]
              tunnel: w3761 -> [_ w3836]
              tunnel: w3760 -> [_ w3814]
              tunnel: w3759 -> [w3782 w3795]
              tunnel: w3758 -> [w3783 w3794]
              tunnel: w3757 -> [_ w3791]
              frame False {
                w3781 = FALSE
                n2244 = Close File(refnum=w3787) -> ()  [unwired: 1 in, 2 out]
                n2245 = case shown="True" w3784 {
                  tunnel: w3785 -> [_ w3789]
                  frame False {
                  }
                  frame True {
                    n2246 = Close File(refnum=w3789) -> ()  [unwired: 1 in, 2 out]
                  }
                }
                n2247 = case shown="True" w3782 {
                  tunnel: w3783 -> [_ w3788]
                  frame False {
                  }
                  frame True {
                    n2248 = Close File(refnum=w3788) -> ()  [unwired: 1 in, 2 out]
                  }
                }
                n2249 = local write "Calibrating Trap..."(w3781) -> ()
                n2250 = call <vilib>:"Beep.vi"() -> ()  [unwired: 3 in, 9 out]
                n2251 = local write "Stop Saving"(w3781) -> ()
                n2252 = property on="Raster Scanning..." class="Bool (strict)"("Val(Sgnl)"=w3781) -> ()  [unwired: 2 in, 2 out]
                "Saving..." <- w3781
              }
              frame True {
                n2253 = local read "Calibrating Trap..."() -> (w3847:bool)
                n2254 = case "Write fl. data" shown="True" w3846 {
                  tunnel: w3845 -> [_ w3881]
                  tunnel: w3844 -> [_ w3880]
                  frame False {
                  }
                  frame True {
                    n2255 = Write to Binary File(file (use dialog)=w3881, data=w3880, 5:FALSE ("prepend array or string size? (T)"), 9:T30."big-endian, network order" ("byte order (0:big-endian, network order)")) -> ()  [unwired: 1 in, 4 out]
                  }
                }
                n2256 = Greater?(x="Save ave N", y=1.0) -> (0:w3850:bool)
                n2257 = Not(x=w3847) -> (.not. x?=w3849:bool)
                n2258 = And(x=w3849, y=w3850) -> (x .and. y?=w3792:bool)
                n2259 = case shown="True" w3792 {
                  tunnel: w3791 -> [w3861 w3872]
                  tunnel: [w3861 w3864] -> w3790
                  tunnel: "Save ave N" -> [_ w3865]
                  frame False {
                  }
                  frame True {
                    w3862 = 2 ("dimension size")
                    n2260 = Array Size(array=w3872) -> (size(s)=w3866:i32)
                    n2261 = Divide(x=w3866, y=w3862) -> (x/y=w3870:dbl)
                    n2262 = Reshape Array(w3872, w3870, w3862) -> (w3871:u64[][])
                    n2263 = Transpose 2D Array(2D array=w3871) -> (transposed array=w3869:u64[][])
                    n2264 = for {
                      tunnel: w3869 -> [w3874] mode=indexing
                      tunnel: [w3873] -> w3863 mode=indexing
                      tunnel: w3865 -> [w3875]
                      workers-P: _ -> [_]
                      n2265 = call "downsample 1D array - U64.vi"("Ave N"=w3875, "Array In"=w3874) -> ("Array Out"=w3873:u64[])  [unwired: 1 in]
                    }
                    n2266 = Transpose 2D Array(2D array=w3863) -> (transposed array=w3868:u64[][])
                    n2267 = Divide(x=w3866, y=w3865) -> (x/y=w3867:dbl)
                    n2268 = Reshape Array(w3868, w3867) -> (w3864:u64[])
                  }
                }
                n2269 = case shown="True" w3792 {
                  tunnel: w3852 -> [w3884 w3896]
                  tunnel: [w3884 w3888] -> w3848
                  tunnel: "Save ave N" -> [_ w3889]
                  tunnel: w3843 -> [_ w3887]
                  frame False {
                    # "don't downsample data for trap calibration"
                  }
                  frame True {
                    n2270 = Array Size(array=w3896) -> (size(s)=w3890:i32)
                    n2271 = Array Size(array=w3887) -> (size(s)=w3886:i32)
                    n2272 = Divide(x=w3890, y=w3886) -> (x/y=w3894:dbl)
                    n2273 = Reshape Array(w3896, w3894, w3886) -> (w3895:i16[][])
                    n2274 = Transpose 2D Array(2D array=w3895) -> (transposed array=w3893:i16[][])
                    n2275 = for {
                      tunnel: w3893 -> [w3899] mode=indexing
                      tunnel: [w3898] -> w3885 mode=indexing
                      tunnel: w3889 -> [w3897]
                      workers-P: _ -> [_]
                      n2276 = call "downsample 1D array - I16.vi"("Ave N"=w3897, "Array In"=w3899) -> ("Array Out"=w3898:i16[])  [unwired: 1 out]
                    }
                    n2277 = Transpose 2D Array(2D array=w3885) -> (transposed array=w3892:i16[][])
                    n2278 = Divide(x=w3890, y=w3889) -> (x/y=w3891:dbl)
                    n2279 = Reshape Array(w3892, w3891) -> (w3888:i16[])
                  }
                }
                n2280 = Index Array(array=w3814, index=1) -> (element=w3817:waveform(dbl))
                n2281 = Index Array(array=w3814, index=0) -> (element=w3819:waveform(dbl))
                n2282 = Unbundle By Name(w3817) -> ("Y"=w3821:dbl[])
                n2283 = Unbundle By Name(w3819) -> ("Y"=w3829:dbl[])
                n2284 = case "Write trap pos. data" shown="True" w3795 {
                  tunnel: w3794 -> [_ w3877]
                  tunnel: w3790 -> [_ w3876]
                  frame False {
                  }
                  frame True {
                    n2285 = Write to Binary File(file (use dialog)=w3877, data=w3876, 5:FALSE ("prepend array or string size? (T)"), 9:T30."big-endian, network order" ("byte order (0:big-endian, network order)")) -> ()  [unwired: 1 in, 4 out]
                  }
                }
                n2286 = Write to Binary File(file (use dialog)=w3855, data=w3848, 5:FALSE ("prepend array or string size? (T)"), 9:T30."big-endian, network order" ("byte order (0:big-endian, network order)")) -> ()  [unwired: 1 in, 4 out]
                n2287 = feedback #26(w3821) -> (w3823:dbl[])
                n2288 = Build Array (concatenate)(w3823, w3821) -> (w3822:dbl[])
                n2289 = Select(t=w3821, s=w3797, f=w3822) -> (s? t:f=w3807:dbl[])
                n2290 = feedback-in #26(w3807) -> ()
                n2291 = feedback #27(w3829) -> (w3842:dbl[])
                n2292 = Build Array (concatenate)(w3842, w3829) -> (w3841:dbl[])
                n2293 = Select(t=w3829, s=w3797, f=w3841) -> (s? t:f=w3816:dbl[])
                n2294 = feedback-in #27(w3816) -> ()
                n2295 = Divide(x=w3856, y=w3857) -> (x/y=w3859:dbl)
                n2296 = Multiply(x=w3859, y=100.0) -> (x*y=w3858:dbl)
                n2297 = Build Array(w3816, w3807) -> (→"Saved APD":dbl[][])
                n2298 = Array Size(array=w3816) -> (size(s)=w3834:i32)
                n2299 = Unbundle By Name(w3836) -> ("Y"=w3840:dbl[])
                n2300 = Subtract(x=w3834, y="N pts to average") -> (x-y=w3810:i32)
                n2301 = Multiply(x="N pts to average", y=u16 2) -> (x*y=w3811:u16)
                n2302 = Subtract(x=w3834, y=w3811) -> (x-y=w3809:i32)
                n2303 = feedback #28(w3840) -> (w3839:dbl[])
                n2304 = Build Array (concatenate)(w3839, w3840) -> (w3838:dbl[])
                n2305 = Select(t=w3840, s=w3797, f=w3838) -> (s? t:f=w3837:dbl[])
                "Trap Delta Graph" <- w3837
                n2306 = feedback-in #28(w3837) -> ()
                n2307 = Array Subset(array=w3816, index=w3810, length="N pts to average") -> (w3833:dbl[])
                n2308 = Array Subset(array=w3816, index=w3809, length="N pts to average") -> (w3832:dbl[])
                n2309 = Array Subset(array=w3807, index=w3810, length="N pts to average") -> (w3813:dbl[])
                n2310 = Array Subset(array=w3807, index=w3809, length="N pts to average") -> (w3812:dbl[])
                n2311 = call-poly <vilib>:"Mean.vi"("X"=w3833) -> ("mean"=w3831:dbl)  [unwired: 1 out]
                n2312 = call-poly <vilib>:"Mean.vi"("X"=w3813) -> ("mean"=w3806:dbl)  [unwired: 1 out]
                n2313 = call-poly <vilib>:"Mean.vi"("X"=w3832) -> ("mean"=w3830:dbl)  [unwired: 1 out]
                n2314 = call-poly <vilib>:"Mean.vi"("X"=w3812) -> ("mean"=w3805:dbl)  [unwired: 1 out]
                n2315 = Subtract(x=w3806, y=w3805) -> (x-y=w3796:dbl)
                "Delta Fl. 2" <- w3796
                n2316 = Subtract(x=w3831, y=w3830) -> (x-y=w3828:dbl)
                "Delta Fl. 1" <- w3828
                n2317 = Initialize Array(w3828, 1 ("dimension size")) -> (w3825:dbl[])
                n2318 = Initialize Array(w3796, 1 ("dimension size")) -> (w3802:dbl[])
                n2319 = feedback #29(w3825) -> (w3826:dbl[])
                n2320 = Build Array (concatenate)(w3826, w3825) -> (w3824:dbl[])
                n2321 = feedback #30(w3802) -> (w3803:dbl[])
                n2322 = Build Array (concatenate)(w3803, w3802) -> (w3801:dbl[])
                n2323 = Select(t=w3825, s=w3797, f=w3824) -> (s? t:f=w3800:dbl[])
                n2324 = feedback-in #29(w3800) -> ()
                n2325 = Select(t=w3802, s=w3797, f=w3801) -> (s? t:f=w3799:dbl[])
                n2326 = feedback-in #30(w3799) -> ()
                n2327 = Build Array(w3800, w3799) -> (→"Save APD Deriv":dbl[][])
              }
            }
            "Progress" <- w3773
            "Progress 2" <- w3773
          }
        }
      }
    }
    n2328 = Divide(x=w2154, y=w2155) -> (x/y=w2145:ext)
    "Trap 2 amplitude" <- w2145
    n2329 = Bundle By Name(cluster=w2408, "Green FB Ch 0"=w2407, "Green FB Ch 1"=w2406) -> (w2392:T49)
